vi "Multiply (Float).vi"(8 "Input Valid":bool=TRUE, 10 "b":fxp<+,32,32>, 11 "a":fxp<+,32,32>) -> (0 "Output Valid":bool, 3 "a*b":fxp<+,32,32>)   [LabVIEW 2012]
doc: "This VI performs single precision multiply on FPGA\n\n\n<b> Latency = 8 Ticks </b>"
uses:
  <vilib>/rvi/IPIntegrationNode/IPINode_Utilities/niFpgaIPINodeSimCore.vi
  <vilib>/rvi/FXPMathLib/basic elements/FxpDiscreteDelay/XNode/nifxpmath_DiscreteDelay.xnode
  <vilib>/rvi/XilinxIP/XIPIN_XNode/niFpgaXIPIN.xnode
  <userlib>/FPGA Library/Code Development/SGL/Multiply Float/Multiply (Float)/FloatMultiply/FloatMultiply_541930154F6B931B952B028B364191DA.dll
  <vilib>/rvi/IPIntegrationNode/IPINode_Xnode/niFpgaIPINode.xnode
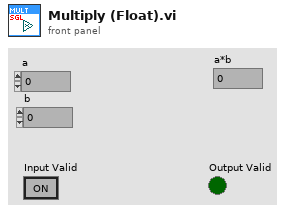
[diagram p1: front panel]
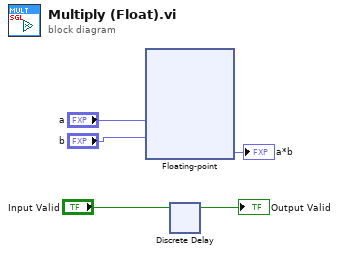
[diagram p0: block diagram]
diagram:
  n1 = xnode ("Floating-point")("a"="a", "b"="b") -> ("result"=→"a*b":fxp<+,32,32>)
  n2 = xnode "Discrete Delay"("D"="Input Valid") -> ("Q"=→"Output Valid":bool)
